vi "tcnChanData.vi"(8 "errorIn":errorcluster, 10 "chanName":string, 11 "TCN":T7) -> (0 "error out":errorcluster caption="errorOut", 2 "outputSignal":T1, 3 "shotNum":string)   [LabVIEW 2017]
uses:
  models/TCN.ctl
  models/Header.ctl
  models/TCN_outputSignal.ctl
  models/TCN_attachedInformation.ctl
  models/TCN_triggerConditions.ctl
  models/TCN_orSignals.ctl
  models/TCN_andSignals.ctl
  models/TCN_pulseClass.ctl
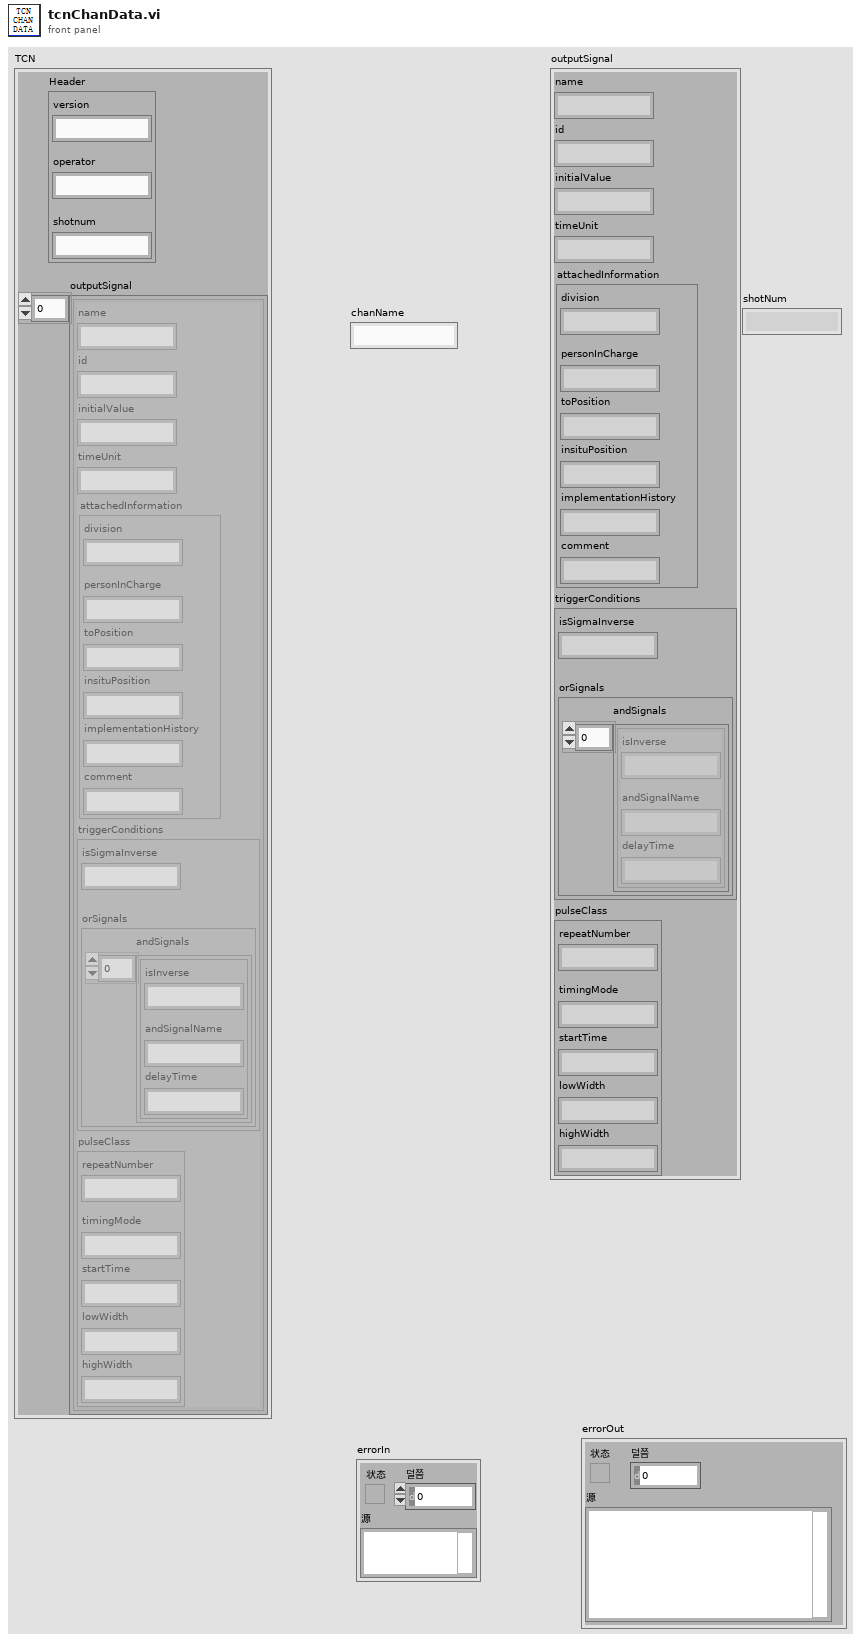
[diagram p1: front panel]
types:
  T1 = typedef "TCN_outputSignal.ctl" = cluster{"name":string, "id":string, "initialValue":string, "timeUnit":string, "attachedInformation":T2, "triggerConditions":T3, "pulseClass":T6}
  T2 = typedef "TCN_attachedInformation.ctl" = cluster{"division":string, "personInCharge":string, "toPosition":string, "insituPosition":string, "implementationHistory":string, "comment":string}
  T3 = typedef "TCN_triggerConditions.ctl" = cluster{"isSigmaInverse":string, "orSignals":T4}
  T4 = typedef "TCN_orSignals.ctl" = cluster{"andSignals":T5[]}
  T5 = typedef "TCN_andSignals.ctl" = cluster{"isInverse":string, "andSignalName":string, "delayTime":string}
  T6 = typedef "TCN_pulseClass.ctl" = cluster{"repeatNumber":string, "timingMode":string, "startTime":string, "lowWidth":string, "highWidth":string}
  T7 = typedef "TCN.ctl" = cluster{"Header":T8, "outputSignal":T1[]}
  T8 = typedef "Header.ctl" = cluster{"version":string, "operator":string, "shotnum":string}
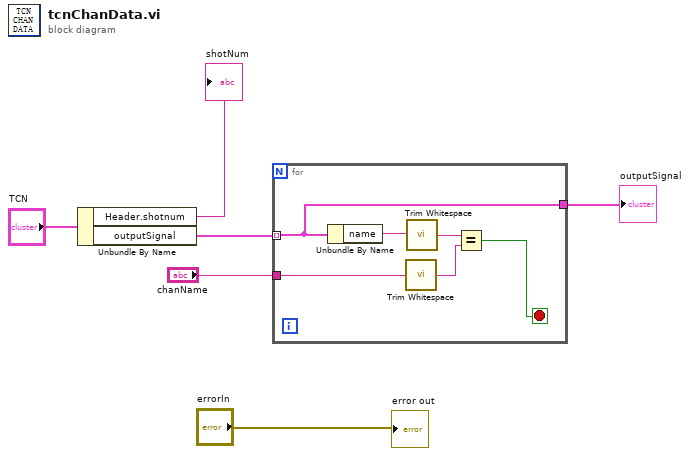
[diagram p0: block diagram]
diagram:
  n1 = Unbundle By Name("TCN") -> ("Header.shotnum"=→"shotNum":string, "outputSignal"=w5:T1[])
  n2 = for {
    tunnel: w5 -> [w7] mode=indexing
    tunnel: "chanName" -> [w11]
    tunnel: [w7] -> w3
    stop <- w8 stop-if-true
    n3 = Unbundle By Name(w7) -> ("name"=w12:string)
    n4 = call <vilib>:"Trim Whitespace.vi"("string"=w11) -> ("trimmed string"=w9:string)  [unwired: 1 in]
    n5 = call <vilib>:"Trim Whitespace.vi"("string"=w12) -> ("trimmed string"=w10:string)  [unwired: 1 in]
    n6 = Equal?(x=w10, y=w9) -> (x = y?=w8:bool)
  }
  "outputSignal" <- w3
  "error out" <- "errorIn"
